vi "Add File to Project.vi"(8 "error in (no error)":errorcluster, 10 "file path":path, 11 "project path":path) -> (0 "error out":errorcluster, 2 "file path dup":path, 3 "project path dup":path)   [LabVIEW 2017]
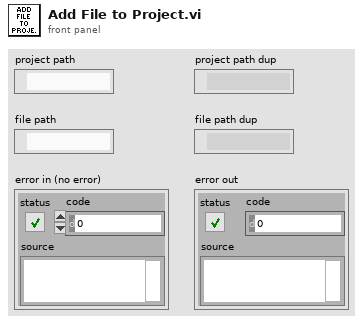
[diagram p1: front panel]
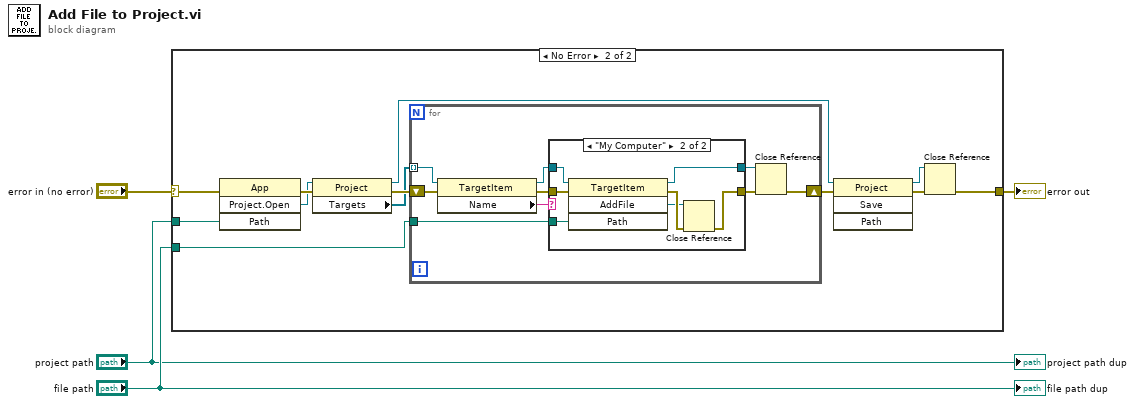
[diagram p0: block diagram]
diagram:
  n1 = case shown="No Error" "error in (no error)" {
    selector: "error in (no error)" -> [w5 w6]
    tunnel: "project path" -> [_ w15]
    tunnel: "file path" -> [_ w12]
    tunnel: [w5 w7] -> w3
    frame Error {
    }
    frame No Error {
      n2 = invoke class="App" method="Project.Open"(error in=w6, "Path"=w15) -> (error out=w16:errorcluster, "Project:Open"=w14:refnum<vi>)  [unwired: 2 in, 2 out]
      n3 = property class="Project"(reference=w14, error in=w16) -> (reference out=w11:refnum<vi>, error out=w17:errorcluster, "Targets"=w13:refnum<vi>[])
      n4 = for {
        tunnel: w13 -> [w21] mode=indexing
        shift-right: [w25] -> w9
        shift-left: w17 -> [w26]
        tunnel: w12 -> [w22]
        n5 = property class="TargetItem"(reference=w21, error in=w26) -> (reference out=w19:refnum<vi>, error out=w18:errorcluster, "Name"=w20:string)
        n6 = case shown="\"My Computer\"" w20 {
          tunnel: [w28 w34] -> w24
          tunnel: [w27 w32] -> w23
          tunnel: w22 -> [_ w31]
          tunnel: w19 -> [w28 w30]
          tunnel: w18 -> [w27 w29]
          frame Default {
          }
          frame "My Computer" {
            n7 = invoke class="TargetItem" method="AddFile"(reference=w30, error in=w29, "Path"=w31) -> (reference out=w34:refnum<vi>, error out=w35:errorcluster, "AddFile"=w33:refnum<vi>)  [unwired: 1 in, 1 out]
            n8 = Close Reference(reference=w33, error in (no error)=w35) -> (error out=w32:errorcluster)
          }
        }
        n9 = Close Reference(reference=w24, error in (no error)=w23) -> (error out=w25:errorcluster)
      }
      n10 = invoke class="Project" method="Save"(reference=w11, error in=w9) -> (reference out=w10:refnum<vi>, error out=w8:errorcluster)  [unwired: 2 in, 2 out]
      n11 = Close Reference(reference=w10, error in (no error)=w8) -> (error out=w7:errorcluster)
    }
  }
  "error out" <- w3
  "project path dup" <- "project path"
  "file path dup" <- "file path"
